vi "Create Default Attributes.vi"(5 "Unique ID":string, 7 "Process Executive Ref":refnum<data-value>, 11 "Stop Under Body Wash in":refnum<class "Stop Under Body Wash.lvclass">) -> (3 "Stop Under Body Wash out":refnum<class "Stop Under Body Wash.lvclass">)   [LabVIEW 2019, in "Stop Under Body Wash.lvclass"]
uses:
  <vilib>/gpm_packages/@cs/Car-wash/Source/Process Steps/Stop Under Body Wash/Stop Under Body Wash.lvclass
  <vilib>/gpm_packages/@cs/test-executive/Source/Test Executive/ITestExecutive/ITest Executive.lvclass
  e7d5f006-14cd-4e15-ad05-c6fb06c04169.vi
  <vilib>/Utility/error.llb/Error Cluster From Error Code.vi
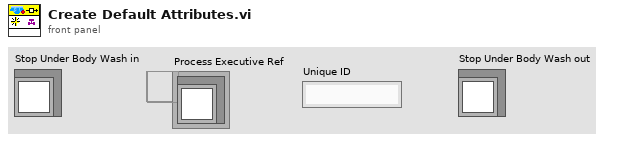
[diagram p1: front panel]
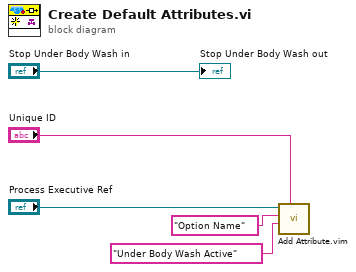
[diagram p0: block diagram]
diagram:
  n1 = call "Add Attribute.vim"("ID"="Unique ID", "Attribute"="Under Body Wash Active" ("Item Name"), "Attribute Name"="Option Name" ("Item Name"), "Test Executive Ref"="Process Executive Ref") -> ()  [unwired: 4 in, 4 out]
  "Stop Under Body Wash out" <- "Stop Under Body Wash in"
